vi "SPI Large.vi"() -> ()   [LabVIEW 2021]
panel:
  out "# Transferred":i32
  in  "# Bytes To Transfer (1+)":i32=4
  out "U8 Array Read":u8[](array[numeric])
  in  "U8 Array Write":u8[](array[numeric])=[170, 240, 170, 240]
  out "Error Message":string
  out "error out":errorcluster
  # "Simple SPI example uses the first found USB device.  You can short MOSI to MISO for testing.  If\nthe number of bytes to transfer is greater than 50, this VI does multiple SPI calls.\n\nMOSI    FIO2\nMISO    FIO3\nCLK      FIO0\nCS        FIO1\n\nIf you short MISO to MOSI, then you will read back the same bytes that you write.  If you short\nMISO to GND, then you will read back zeros.  If you short MISO to VS or leave it\nunconnected, you will read back 255s.\n\nTested with UD V2.77, U3 firmware V1.44, and UE9 firmware 1.40/1.84 (Comm/Control).  Will\nhave to change to FIO4-7 on a U3-HV."
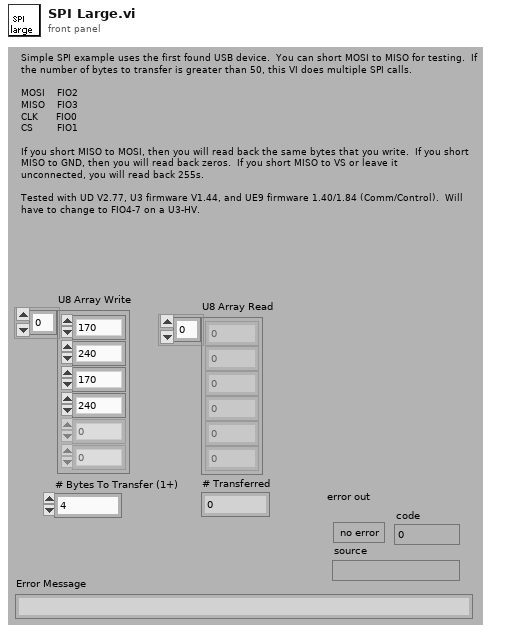
[diagram p1: front panel]
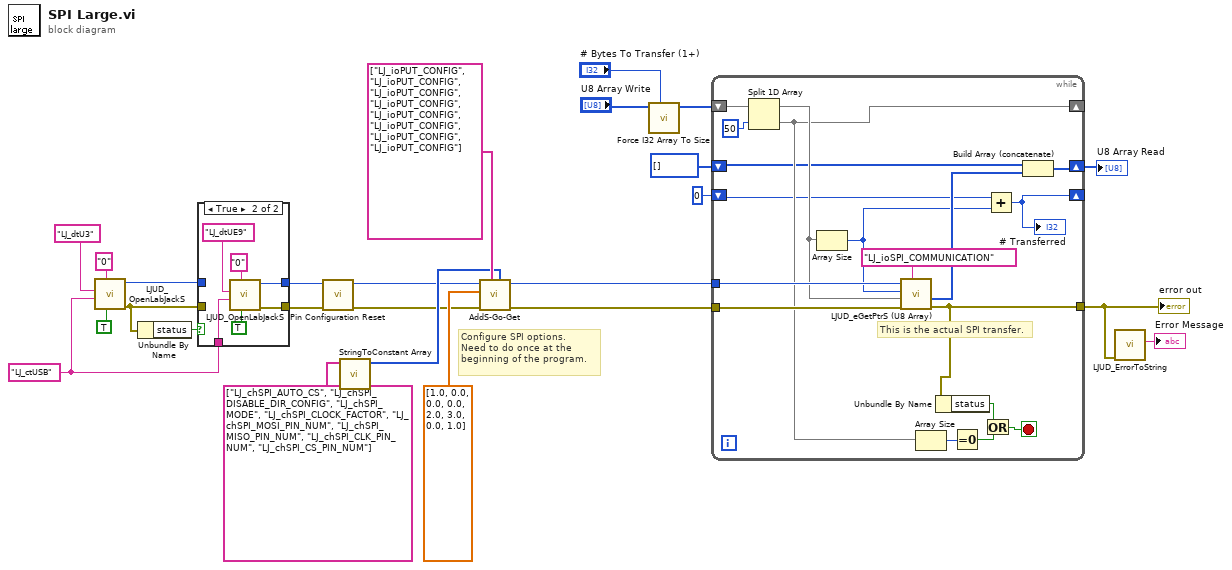
[diagram p0: block diagram]
diagram:
  w3 = "LJ_ctUSB" ("ConnectionType")
  # "Configure SPI options.\nNeed to do once at the\nbeginning of the program."
  n1 = call "LJUD_OpenLabJackS.vi"("FirstFound"=TRUE, "Address"="0", "ConnectionType"=w3, "DeviceType"="LJ_dtU3") -> ("error out"=w5:errorcluster, "Handle"=w4:i32)  [unwired: 5 in, 1 out]
  n2 = Unbundle By Name(w5) -> ("status"=w6:bool)
  n3 = case shown="True" w6 {
    tunnel: w5 -> [w27 _]
    tunnel: [w27 w30] -> w1
    tunnel: w4 -> [w26 _]
    tunnel: [w26 w29] -> w2
    tunnel: w3 -> [_ w31]
    frame False {
    }
    frame True {
      n4 = call "LJUD_OpenLabJackS.vi"("FirstFound"=TRUE, "Address"="0", "ConnectionType"=w31, "DeviceType"="LJ_dtUE9") -> ("error out"=w30:errorcluster, "Handle"=w29:i32)  [unwired: 5 in, 1 out]
    }
  }
  n5 = call "Pin Configuration Reset.vi"("error in"=w1, "Handle In"=w2) -> ("error out"=w16:errorcluster, "Handle Out"=w15:i32)  [unwired: 8 in]
  n6 = call "StringToConstant Array.vi"("String Constant Array In"=string[] ["LJ_chSPI_AUTO_CS", "LJ_chSPI_DISABLE_DIR_CONFIG", "LJ_chSPI_MODE", "LJ_chSPI_CLOCK_FACTOR", "LJ_chSPI_MOSI_PIN_NUM", "LJ_chSPI_MISO_PIN_NUM", "LJ_chSPI_CLK_PIN_NUM", "LJ_chSPI_CS_PIN_NUM"] ("IOTypes")) -> ("I32 Constant Array Out"=w20:i32[])  [unwired: 10 in]
  n7 = call "AddS-Go-Get.vi"("Channels"=w20, "IOTypes"=string[] ["LJ_ioPUT_CONFIG", "LJ_ioPUT_CONFIG", "LJ_ioPUT_CONFIG", "LJ_ioPUT_CONFIG", "LJ_ioPUT_CONFIG", "LJ_ioPUT_CONFIG", "LJ_ioPUT_CONFIG", "LJ_ioPUT_CONFIG"], "error in"=w16, "Values Write"=dbl[] [1.0, 0.0, 0.0, 0.0, 2.0, 3.0, 0.0, 1.0], "Handle In"=w15) -> ("error out"=w19:errorcluster, "Handle Out"=w18:i32)  [unwired: 4 in, 1 out]
  n8 = call "Force I32 Array To Size.vi"("# Elements"="# Bytes To Transfer (1+)", "I32 Array In"="U8 Array Write") -> ("I32 Array Out"=w13:i32[])  [unwired: 9 in]
  n9 = while {
    shift-left: 0 -> [w34]
    shift-right: [w35] -> _
    shift-left: u8[] [] ("U8 Array Read") -> [w39]
    shift-right: [w37] -> w11
    shift-left: w13 -> [w48]
    shift-right: [w40] -> _
    tunnel: w18 -> [w49]
    tunnel: w19 -> [w50]
    tunnel: [w43] -> w25
    stop <- w46 stop-if-true
    # "This is the actual SPI transfer."
    n10 = Split 1D Array(array=w48, index=50) -> (first subarray=w45:i32[], second subarray=w40:i32[])
    n11 = Array Size(array=w45) -> (size(s)=w36:i32)
    n12 = call "LJUD_eGetPtrS (U8 Array).vi"("IOType"="LJ_ioSPI_COMMUNICATION", "error in"=w50, "U8 Array Write"=w45, "Value"=w36, "Handle In"=w49) -> ("error out"=w43:errorcluster, "U8 Array Read"=w38:u8[])  [unwired: 3 in, 2 out]
    n13 = Array Size(array=w40) -> (size(s)=w44:i32)
    n14 = Unbundle By Name(w43) -> ("status"=w42:bool)
    n15 = Equal To 0?(x=w44) -> (x = 0?=w41:bool)
    n16 = Or(x=w42, y=w41) -> (x .or. y?=w46:bool)
    n17 = Add(x=w34, y=w36) -> (x+y=w35:i32)
    "# Transferred" <- w35
    n18 = Build Array (concatenate)(w39, w38) -> (w37:u8[])
  }
  "error out" <- w25
  "U8 Array Read" <- w11
  n19 = call "LJUD_ErrorToString.vi"("error in"=w25) -> ("String"=→"Error Message":string)  [unwired: 10 in]
